vi "Read TPDO.vi"() -> ()   [LabVIEW 2016]
uses:
  <vilib>/CANopenLib/CANOPEN.llb/CANopen TPDO Create.vi
  <vilib>/CANopenLib/CANOPEN.llb/CANopen TPDO Start.vi
  <vilib>/CANopenLib/CANOPEN.llb/CANopen TPDO Stop.vi
  <vilib>/CANopenLib/CANOPEN.llb/CANopen TPDO Close.vi
  <vilib>/CANopenLib/CANOPEN.llb/CANopen Interface Close.vi
panel:
  in  "PDO channel":u8(ring) items=["PDO 1", "PDO 2", "PDO 3", "PDO 4"]
  in  "COB-ID (0)":u32
  in  "Node ID":u8 min=1 max=127 step=1
  out "data":u8[](array[numeric])
  out "error out":errorcluster
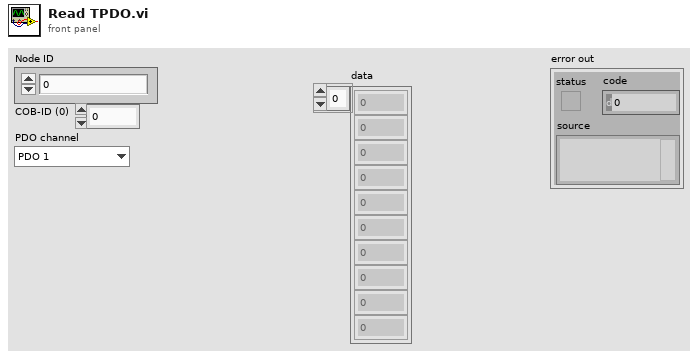
[diagram p1: front panel]
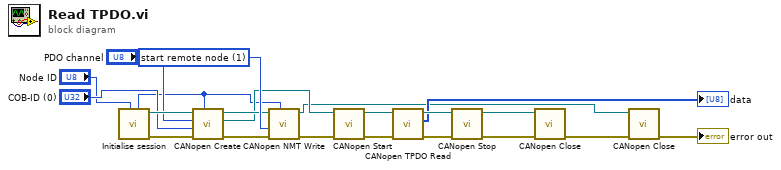
[diagram p0: block diagram]
diagram:
  w10 = u16 1 items=["start remote node"=1, "stop remote node"=2, "enter pre-operational"=128, "reset node"=129, "reset communication"=130] ("command")
  n1 = call "Initialise session.vi"("Node ID"="Node ID") -> ("error out"=w20:errorcluster, "interface object out"=w21:refnum<k20>, "Used Node ID"=w1:u8)  [unwired: 8 in]
  n2 = call-poly <vilib>:"CANopen Create.vi"("node-ID"=w1, "error in (no error)"=w20, "COB-ID (0)"="COB-ID (0)", "PDO channel"="PDO channel", "interface object in"=w21) -> ("error out"=w7:errorcluster, "TPDO object out"=w3:refnum<k20>, "interface object out"=w4:refnum<k20>)  [unwired: 4 in]
  n3 = call <vilib>:"CANopen NMT Write.vi"("node-ID (0)"=w1, "error in (no error)"=w7, "command"=w10, "interface object in"=w4) -> ("error out"=w6:errorcluster, "interface object out"=w2:refnum<k20>)  [unwired: 6 in]
  n4 = call-poly <vilib>:"CANopen Start.vi"("error in (no error)"=w6, "TPDO object in"=w3) -> ("error out"=w5:errorcluster, "TPDO object out"=w9:refnum<k20>)  [unwired: 8 in]
  n5 = call <vilib>:"CANopen TPDO Read.vi"("error in (no error)"=w5, "TPDO object in"=w9) -> ("error out"=w18:errorcluster, "data"=→"data":u8[], "TPDO object out"=w19:refnum<k20>)  [unwired: 5 in, 2 out]
  n6 = call-poly <vilib>:"CANopen Stop.vi"("error in (no error)"=w18, "TPDO object in"=w19) -> ("error out"=w16:errorcluster, "TPDO object out"=w17:refnum<k20>)  [unwired: 8 in]
  n7 = call-poly <vilib>:"CANopen Close.vi"("error in (no error)"=w16, "TPDO object in"=w17) -> ("error out"=w15:errorcluster)  [unwired: 9 in]
  n8 = call-poly <vilib>:"CANopen Close.vi"("error in (no error)"=w15, "interface object in"=w2) -> ("error out"=→"error out":errorcluster)  [unwired: 9 in]
